vi "2x3CIM Set Output.vi"(8 "error in":errorcluster, 9 "RightMotorsSpeed":dbl, 10 "LeftMotorsSpeed":dbl) -> (0 "error out":errorcluster)   [LabVIEW 2015]
doc: "Sets output to dual VexPro 3-CIM drive assemblies."
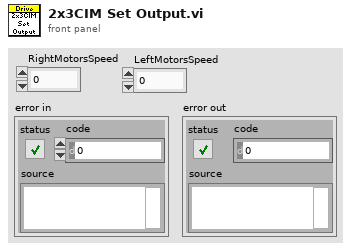
[diagram p1: front panel]
types:
  T1 = typedef "WPI_MotorControlDeviceRef.ctl" = cluster{"DeviceStatus":errorcluster, "Type":T2, "PWM":cluster{"PWM Channel":T3, "DeadBand":T4}, "CAN":cluster{"Device Number":u8, "Control Mode":T5, "Semaphore":T6, "Max Vout":dbl, "TalonSRX Control Mode":T7}, "Invert":bool}
  T2 = typedef "WPI_MotorControlType.ctl" = enum16{"PWM", "CAN", "CANTalonSRX"}
  T3 = typedef "FPGA_DIOPWMChannel.ctl" = enum8{"PWM 0", "PWM 1", "PWM 2", "PWM 3", "PWM 4", "PWM 5", "PWM 6", "PWM 7", "PWM 8", "PWM 9", "PWM MXP 0", "PWM MXP 1", "PWM MXP 2", "PWM MXP 3", "PWM MXP 4", "PWM MXP 5", "PWM MXP 6", "PWM MXP 7", "PWM MXP 8", "PWM MXP 9", "Invalid"}
  T4 = typedef "WPI_PWMDeadband.ctl" = cluster{"Name":string, "maxPositivePwm":i32, "minPositivePwm":i32, "centerPwm":i32, "maxNegativePwm":i32, "minNegativePwm":i32, "angularRange":u16}
  T5 = typedef "WPI_CANJaguar_ControlMode.ctl" = enum8{"Percent VBus", "Current", "Speed", "Position", "Voltage"}
  T6 = typedef "Semaphore RefNum" = refnum<k1>
  T7 = typedef "WPI_CANTalonSRX_APIControlMode.ctl" = enum8{"Percent VBus", "Speed", "Position", "Slave", "Unchanged / Invalid", "Voltage Compensation", "Current", "Motion Profile"}
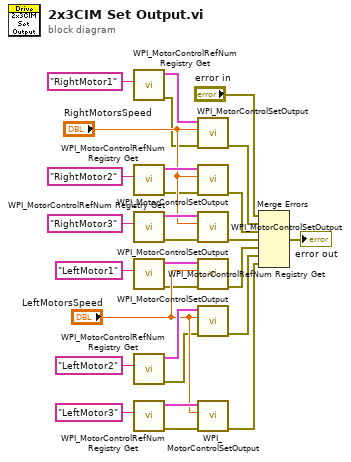
[diagram p0: block diagram]
diagram:
  n1 = call <vilib>:"WPI_MotorControlRefNum Registry Get.vi"("refnum name"="RightMotor1") -> ("error out"=w9:errorcluster, "MotorControlDevRef"=w28:T1)  [unwired: 9 in]
  n2 = call <vilib>:"WPI_MotorControlRefNum Registry Get.vi"("refnum name"="RightMotor2") -> ("error out"=w10:errorcluster, "MotorControlDevRef"=w25:T1)  [unwired: 9 in]
  n3 = call <vilib>:"WPI_MotorControlRefNum Registry Get.vi"("refnum name"="RightMotor3") -> ("error out"=w11:errorcluster, "MotorControlDevRef"=w27:T1)  [unwired: 9 in]
  n4 = call <vilib>:"WPI_MotorControlRefNum Registry Get.vi"("refnum name"="LeftMotor1") -> ("error out"=w12:errorcluster, "MotorControlDevRef"=w22:T1)  [unwired: 9 in]
  n5 = call <vilib>:"WPI_MotorControlRefNum Registry Get.vi"("refnum name"="LeftMotor2") -> ("error out"=w13:errorcluster, "MotorControlDevRef"=w19:T1)  [unwired: 9 in]
  n6 = call <vilib>:"WPI_MotorControlRefNum Registry Get.vi"("refnum name"="LeftMotor3") -> ("error out"=w14:errorcluster, "MotorControlDevRef"=w21:T1)  [unwired: 9 in]
  n7 = call <vilib>:"WPI_MotorControlSetOutput.vi"("error in (no error)"=w9, "Output"="RightMotorsSpeed", "MotorControlDevRef"=w28) -> ("error out"=w8:errorcluster)  [unwired: 6 in, 2 out]
  n8 = call <vilib>:"WPI_MotorControlSetOutput.vi"("error in (no error)"=w10, "Output"="RightMotorsSpeed", "MotorControlDevRef"=w25) -> ("error out"=w7:errorcluster)  [unwired: 6 in, 2 out]
  n9 = call <vilib>:"WPI_MotorControlSetOutput.vi"("error in (no error)"=w11, "Output"="RightMotorsSpeed", "MotorControlDevRef"=w27) -> ("error out"=w6:errorcluster)  [unwired: 6 in, 2 out]
  n10 = call <vilib>:"WPI_MotorControlSetOutput.vi"("error in (no error)"=w12, "Output"="LeftMotorsSpeed", "MotorControlDevRef"=w22) -> ("error out"=w5:errorcluster)  [unwired: 6 in, 2 out]
  n11 = call <vilib>:"WPI_MotorControlSetOutput.vi"("error in (no error)"=w13, "Output"="LeftMotorsSpeed", "MotorControlDevRef"=w19) -> ("error out"=w4:errorcluster)  [unwired: 6 in, 2 out]
  n12 = call <vilib>:"WPI_MotorControlSetOutput.vi"("error in (no error)"=w14, "Output"="LeftMotorsSpeed", "MotorControlDevRef"=w21) -> ("error out"=w3:errorcluster)  [unwired: 6 in, 2 out]
  n13 = Merge Errors("error in", w8, w7, w6, w5, w4, w3) -> (→"error out":errorcluster)
